vi "Cleanup.vi"(8 "error in (no error)":errorcluster, 11 "FileStream in":refnum<class "FileStream.lvclass">) -> (0 "error out":errorcluster, 3 "FileStream out":refnum<class "FileStream.lvclass">)   [LabVIEW 2020, in "IO.lvlib" / "FileStream.lvclass"]
uses:
  FileStream.lvclass
  FileStream.lvclass/FileStream.ctl
  Stream/Stream.lvclass
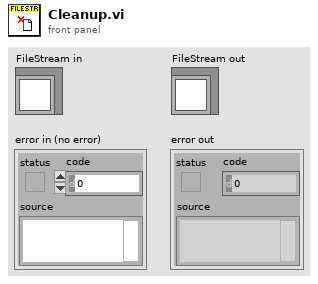
[diagram p1: front panel]
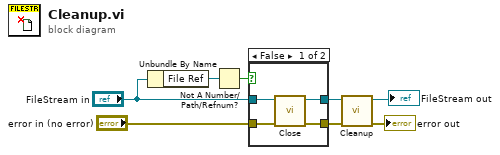
[diagram p0: block diagram]
diagram:
  n1 = Unbundle By Name("FileStream in") -> ("File Ref"=w4:refnum<file>)
  n2 = Not A Number/Path/Refnum?(number/path/refnum=w4) -> (NaN/Path/Refnum?=w3:bool)
  n3 = case shown="False" w3 {
    tunnel: "FileStream in" -> [w12 w14]
    tunnel: "error in (no error)" -> [w11 w13]
    tunnel: [w10 w13] -> w6
    tunnel: [w9 w14] -> w5
    frame False {
      n4 = call-dynamic "Close.vi"("error in (no error)"=w11, "FileStream in"=w12) -> ("error out"=w10:errorcluster, "FileStream out"=w9:refnum<class "FileStream.lvclass">)  [unwired: 8 in]
    }
    frame True {
    }
  }
  n5 = call-parent "Cleanup.vi"("error in (no error)"=w6, "Stream in"=w5) -> ("error out"=→"error out":errorcluster, "Stream out"=→"FileStream out":refnum<class "FileStream.lvclass">)  [unwired: 8 in]
